vi "LEBITplc.UpdateLLF.vi"(0 "i ref in":refnum<vi>, 2 "file path (use dialog)":path, 3 "FileName":string, 4 "GUI Name":string, 5 "error in":errorcluster, 7 "LoadorSave":i16, 9 "Log":bool) -> (14 "i ref in":refnum<vi>, 19 "error out":errorcluster)   [LabVIEW 2014, in "LEBITplc.lvlib"]
uses:
  LEBITplc.lvlib
  CSlibraries/UtilityLib/UtilityLib.valueStatus.ctl
  CSCore/CSSystem/CoreDefs/CoreDefs.error_type.ctl
  CSCore/CSSystem/CoreDefs/CoreDefs.error_severity.ctl
  CSlibraries-extern/DimLVEvent/LVDimInterface/LVDimInterface.lvlib
  CSCore/CSSystem/CoreLib/CoreLib.lvlib
  CSlibraries/UtilityLib/UtilityLib.lvlib
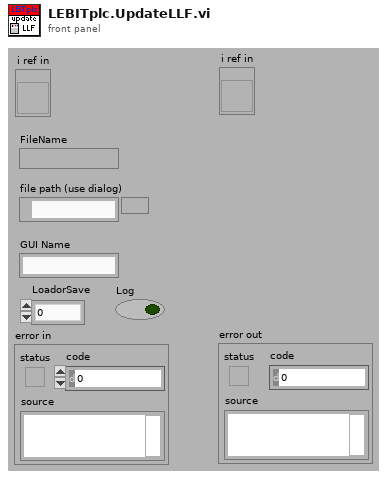
[diagram p1: front panel]
types:
  T1 = typedef "UtilityLib.lvlib/UtilityLib.valueStatus.ctl" = enum16{"no info available", "stand by/off", "on", "warning", "alarm/malfunction", "not implemented", "user action required", "important information", "system default", "control default", "indicator default", "button default"}
  T2 = typedef "CoreDefs.error_severity.ctl" = enum16{"undefined", "information", "warning", "error", "fatal"}
  T3 = typedef "CoreDefs.error_type.ctl" = enum16{"no error", "can't load process", "can't unload process", "process does not exist", "can't install process", "can't remove process", "unknown function", "time out", "can't execute function", "duplicate queue name", "super not found", "caller queue invalid", "can't ping process", "unknown error", "VISA Error", "VISA timeout", "GPIB timeout", "GPIB error", "communication error", "data type mismatch", "can't read data from OPC server", "can't write data to OPC server", "OET error", "function not implemented", "process already exists", "invalid Shared Variable name", "error writing Shared Variable", "error reading Shared Variable", "invalid client name", "corrupt database", "unknown class", "call not authorized", "parameter out of range", "OET timeout: can't get data to modify", "invalid queue name", "requested operation incompatible with current state", "event undefined", "event disabled", "state undefined", "caller is not a friend", "EventBuilder: bad eventID", "EventBuilder: no DAQ devices", "a thread must not stop itself", "UNUSED ELEMENT4", "DiscArchiver: eventData incomplete", "DiscArchiver: eventData does not belong to run", "DiscArchiver: can't open file", "DiscArchiver: can't write to file", "DiscArchiver: available disc space low", "can't acquire semaphore", "error reading data from database", "notifier object is not existing", "can't register process", "can't unregister process", "illegal event type", "object disabled", "object already exists", "can't change state", "Instrument not found", "no connection to remote node", "invalid reference", "N/A", "UNUSED ELEMENT 1", "element not found", "illegal TCP/IP connection detected", "object does not exist", "invalid access ID", "unknown CS system", "invalid privilige", "unsupported data type", "unsupported server type", "IO server already exists", "Shared Variable already exists"}
  T4 = typedef "LEBITplc.lvlib/LEBITplc.i attribute.ctl" = cluster{"LLFLocation":string, "SetFileLocation":string, "nickNames":string[], "setValuePLCServiceID":i32[], "GUIServiceID":i32[], "monValuePLC":string[], "SetValueServiceID":i32[], "MonValueServiceID":i32[], "SetValue":dbl[][], "SetValueMin":dbl[], "SetValueMax":dbl[], "SetValueInfoServiceID":i32[], "GUINames":string[], "ListOfBases":string[], "Scale":dbl[], "Offset":dbl[], "setValuePLC":string[], "BaseName":string[], "ScaleServiceID":i32[], "OffsetServiceID":i32[], "AllPLCValues":string[], "CondSpecialArray":string[][], "CondSpecialIndex":i32[], "CondSpecialMonValue":dbl[], "RecentlyChanged":i32[], "SetFileLocationID":i32, "Dependent-Monitors":string[][], "LastLoadedFiles":string[], "IonGuideCalibLocation":string, "Monitor Dependent":string[], "Special":string[], "PLC?":bool[], "Start Date":string, "ListOfBasesServiceID":i32, "SETRA VISA resource":refnum<visa-resource-name>}
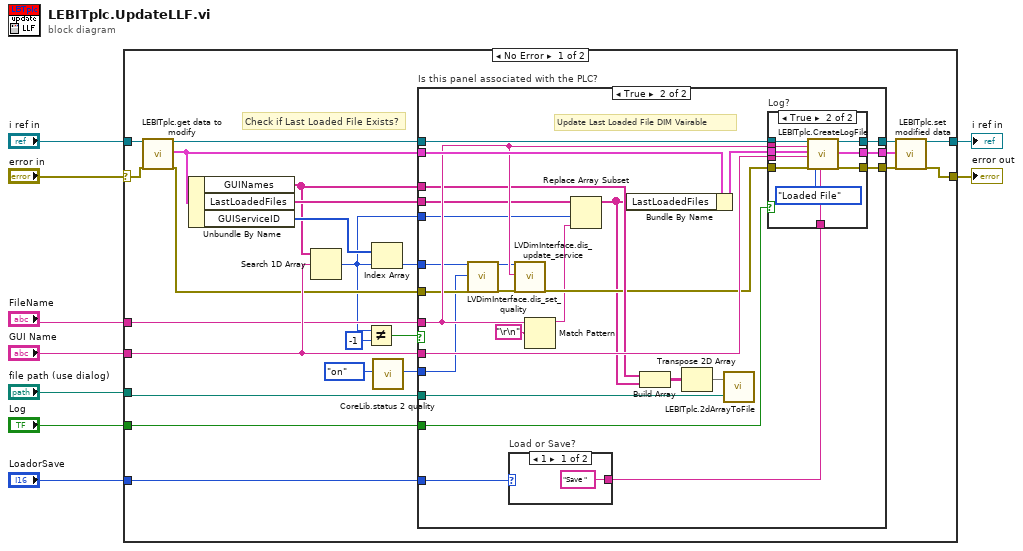
[diagram p0: block diagram]
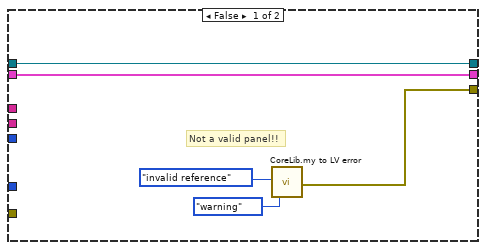
[diagram p2: hidden frame]
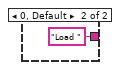
[diagram p3: hidden frame]
diagram:
  n1 = case shown="No Error" "error in" {
    selector: "error in" -> [w28 w80]
    tunnel: "GUI Name" -> [w27 _]
    tunnel: "i ref in" -> [w33 w81]
    tunnel: [w31 w81] -> w7
    tunnel: [w30 w80] -> w9
    tunnel: "FileName" -> [w25 _]
    tunnel: "file path (use dialog)" -> [w26 _]
    tunnel: "Log" -> [w11 _]
    tunnel: "LoadorSave" -> [w10 _]
    frame No Error {
      # "Check if Last Loaded File Exists?"
      n2 = call "LEBITplc.get data to modify.vi"("i ref in"=w33, "error in (no error)"=w28) -> ("i ref out"=w29:refnum<vi>, "i attribute"=w32:T4, "error out"=w21:errorcluster)  [unwired: 14 in, 1 out]
      n3 = Unbundle By Name(w32) -> ("GUINames"=w14:string[], "LastLoadedFiles"=w15:string[], "GUIServiceID"=w24:i32[])
      n4 = Search 1D Array(1D array=w14, element=w27) -> (index of element=w19:i32)  [unwired: 1 in]
      n5 = Not Equal?(x=w19, y=-1) -> (x != y?=w22:bool)
      n6 = Index Array(array=w24, index=w19) -> (element=w20:i32)
      n7 = call "CoreLib.status 2 quality.vi"("valueStatus"=UtilityLib.valueStatus."on") -> ("quality"=w13:i32)  [unwired: 18 in]
      n8 = case "Is this panel associated with the PLC?" shown="True" w22 {
        tunnel: w32 -> [w37 w63]
        tunnel: w29 -> [w38 w62]
        tunnel: w14 -> [_ w54]
        tunnel: w27 -> [_ w61]
        tunnel: w26 -> [_ w64]
        tunnel: w25 -> [_ w60]
        tunnel: w19 -> [_ w56]
        tunnel: w20 -> [_ w44]
        tunnel: w21 -> [_ w43]
        tunnel: [w37 w59] -> w18
        tunnel: [w38 w58] -> w17
        tunnel: [w34 w57] -> w16
        tunnel: w15 -> [_ w55]
        tunnel: w13 -> [_ w42]
        tunnel: w11 -> [_ w41]
        tunnel: w10 -> [_ w40]
        frame False {
          # "Not a valid panel!!"
          n9 = call "CoreLib.my to LV error.vi"("ErrorTypes"=CoreDefs.error_type."invalid reference", "severityLevel"=CoreDefs.error_severity."warning") -> ("myErrorCluster"=w34:errorcluster)  [unwired: 16 in, 1 out]
        }
        frame True {
          # "Update Last Loaded File DIM Vairable"
          n10 = call "LVDimInterface.dis_set_quality.vi"("my_serviceID"=w44, "quality"=w42, "error in (no error)"=w43) -> ("my_serviceID (out)"=w46:i32, "error out"=w45:errorcluster)  [unwired: 15 in]
          n11 = case "Load or Save?" shown="1" w40 {
            tunnel: ["Save " "Load "] -> w39
            frame 1 {
            }
            frame 0, Default {
            }
          }
          n12 = call "LVDimInterface.dis_update_service.vi"("my_serviceID"=w46, "data"=w60, "error in (no error)"=w45) -> ("error out"=w53:errorcluster)  [unwired: 14 in, 2 out]
          n13 = Match Pattern(string=w60, regular expression="\r\n") -> (before substring=w51:string)  [unwired: 1 in, 3 out]
          n14 = Replace Array Subset(array=w55, new element=w51, index=w56) -> (w49:string[])
          n15 = Bundle By Name(cluster=w63, "LastLoadedFiles"=w49) -> (w52:T4)
          n16 = Build Array(w54, w49) -> (w48:string[][])
          n17 = Transpose 2D Array(2D array=w48) -> (transposed array=w47:string[][])
          n18 = call "LEBITplc.2dArrayToFile.vi"("file path (dialog if empty)"=w64, "Array"=w47) -> ()  [unwired: 2 in]
          n19 = case "Log?" shown="True" w41 {
            tunnel: w62 -> [w69 w79]
            tunnel: w61 -> [_ w78]
            tunnel: w60 -> [_ w77]
            tunnel: [w68 w76] -> w59
            tunnel: [w69 w75] -> w58
            tunnel: [w67 w74] -> w57
            tunnel: w53 -> [w67 w73]
            tunnel: w52 -> [w68 w71]
            tunnel: w39 -> [_ w70]
            frame False {
            }
            frame True {
              n20 = call "LEBITplc.CreateLogFile.vi"("i ref in"=w79, "File Name"=w77, "i attribute in"=w71, "nickName"=w78, "error in"=w73, "Enum"=enum16{"Set Value", "Loaded File"}."Loaded File", "LoadOrSave"=w70) -> ("i ref out"=w75:refnum<vi>, "i attribute out"=w76:T4, "error out"=w74:errorcluster)  [unwired: 10 in]
            }
          }
        }
      }
      n21 = call "LEBITplc.set modified data.vi"("i ref in"=w17, "i attribute"=w18, "error in (no error)"=w16) -> ("i ref out"=w31:refnum<vi>, "error out"=w30:errorcluster)  [unwired: 15 in]
    }
    frame Error {
    }
  }
  "error out" <- w9
  "i ref in" <- w7
